vi "R5DOControl.vi"(8 "error constant":errorcluster, 11 "LabVIEW Web Service":refnum<class "Web Service.lvclass">) -> ()   [LabVIEW 2016]
uses:
  <vilib>/wsapi/Web Service.lvclass
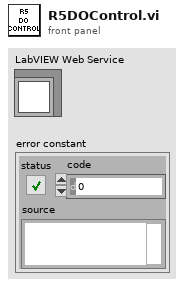
[diagram p1: front panel]
types:
  T1 = cluster{"DO Set Point":dbl, "Pump Time On, secs":dbl}
  T2 = cluster{"Signal, mA":dbl, "Value, UNITS HERE":dbl}
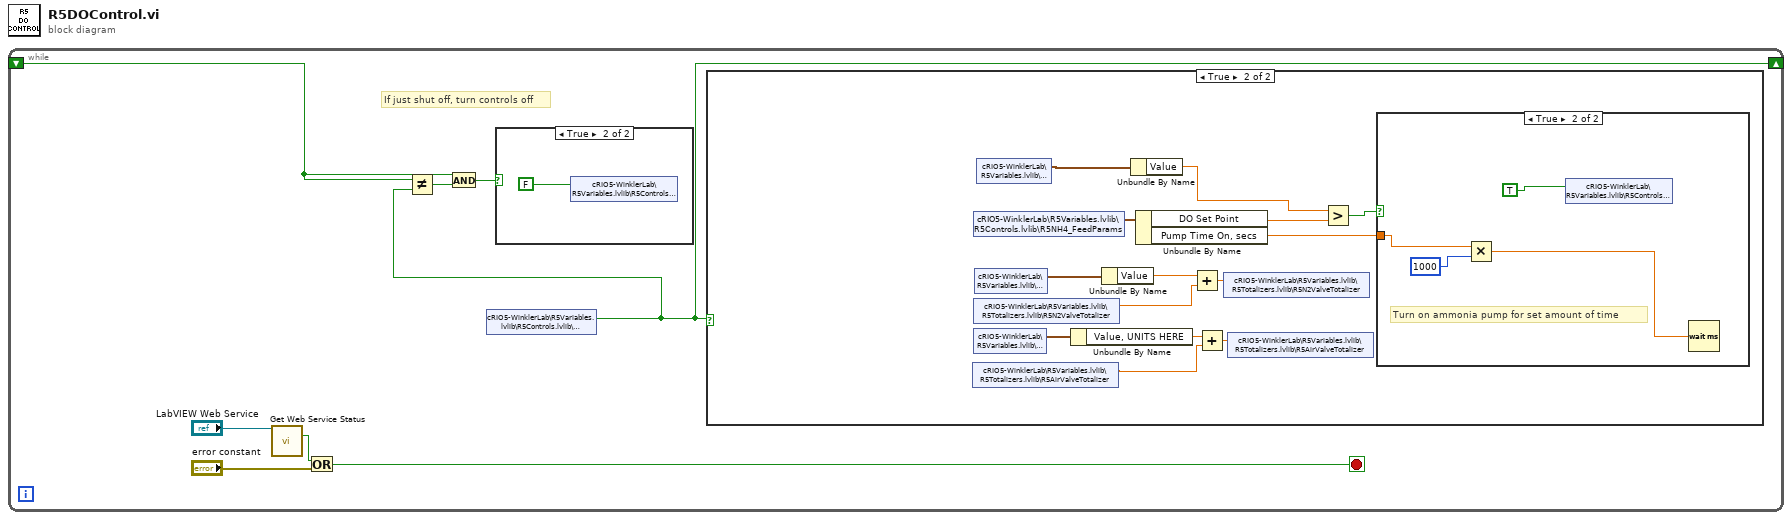
[diagram p0: block diagram]
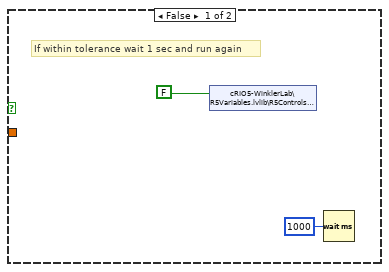
[diagram p4: hidden frame]
diagram:
  n1 = while {
    shift-right: [w1] -> _
    shift-left: _ -> [w2]
    stop <- w5 stop-if-true
    # "If just shut off, turn controls off"
    n2 = call <vilib>:"Get Web Service Status.vi"("LabVIEW Web Service"="LabVIEW Web Service") -> ("service stopping?"=w8:bool)  [unwired: 12 in, 2 out]
    n3 = Or(x=w8, y="error constant") -> (x .or. y?=w5:bool)
    n4 = shared-variable "cRIO5-WinklerLab\\R5Variables.lvlib\\R5Controls.lvlib\\R5DOSwitch"() -> (w1:bool)  [unwired: 1 in, 1 out]
    n5 = Not Equal?(x=w2, y=w1) -> (x != y?=w3:bool)
    n6 = And(x=w2, y=w3) -> (x .and. y?=w4:bool)
    n7 = case shown="True" w4 {
      frame False {
      }
      frame True {
        n8 = shared-variable "cRIO5-WinklerLab\\R5Variables.lvlib\\R5Controls.lvlib\\R5NH4Feed"(FALSE) -> ()  [unwired: 1 in, 1 out]
      }
    }
    n9 = case shown="True" w1 {
      frame False {
        # "Don't do anything if control is off"
      }
      frame True {
        n10 = shared-variable "cRIO5-WinklerLab\\R5Variables.lvlib\\R5Totalizers.lvlib\\R5AirValveTotalizer"() -> (w17:dbl)  [unwired: 1 in, 1 out]
        n11 = shared-variable "cRIO5-WinklerLab\\R5Variables.lvlib\\R5Controls.lvlib\\R5NH4_FeedParams"() -> (w13:T1)  [unwired: 1 in, 1 out]
        n12 = shared-variable "cRIO5-WinklerLab\\R5Variables.lvlib\\R5Totalizers.lvlib\\R5N2ValveTotalizer"() -> (w16:dbl)  [unwired: 1 in, 1 out]
        n13 = shared-variable "cRIO5-WinklerLab\\R5Variables.lvlib\\R5Signals.lvlib\\R5Air"() -> (w18:T2)  [unwired: 1 in, 1 out]
        n14 = shared-variable "cRIO5-WinklerLab\\R5Variables.lvlib\\R5Signals.lvlib\\R5N2"() -> (w19:cluster{"Signal":dbl, "Value":dbl})  [unwired: 1 in, 1 out]
        n15 = shared-variable "cRIO5-WinklerLab\\R5Variables.lvlib\\R5Signals.lvlib\\R5DO"() -> (w20:cluster{"Signal":dbl, "Value":dbl})  [unwired: 1 in, 1 out]
        n16 = Unbundle By Name(w18) -> ("Value, UNITS HERE"=w22:dbl)
        n17 = Unbundle By Name(w19) -> ("Value"=w21:dbl)
        n18 = Unbundle By Name(w20) -> ("Value"=w11:dbl)
        n19 = Unbundle By Name(w13) -> ("DO Set Point"=w12:dbl, "Pump Time On, secs"=w10:dbl)
        n20 = Add(x=w21, y=w16) -> (x+y=w15:dbl)
        n21 = Add(x=w22, y=w17) -> (x+y=w14:dbl)
        n22 = shared-variable "cRIO5-WinklerLab\\R5Variables.lvlib\\R5Totalizers.lvlib\\R5N2ValveTotalizer"(w15) -> ()  [unwired: 1 in, 1 out]
        n23 = shared-variable "cRIO5-WinklerLab\\R5Variables.lvlib\\R5Totalizers.lvlib\\R5AirValveTotalizer"(w14) -> ()  [unwired: 1 in, 1 out]
        n24 = Greater?(x=w11, y=w12) -> (0:w23:bool)
        n25 = case shown="True" w23 {
          tunnel: w10 -> [_ w28]
          frame False {
            # "If within tolerance wait 1 sec and run again"
            n26 = shared-variable "cRIO5-WinklerLab\\R5Variables.lvlib\\R5Controls.lvlib\\R5NH4Feed"(FALSE) -> ()  [unwired: 1 in, 1 out]
            n27 = Wait (ms)(milliseconds to wait=u32 1000) -> ()  [unwired: 1 out]
          }
          frame True {
            # "Turn on ammonia pump for set amount of time"
            n28 = Multiply(x=w28, y=1000) -> (x*y=w27:dbl)
            n29 = shared-variable "cRIO5-WinklerLab\\R5Variables.lvlib\\R5Controls.lvlib\\R5NH4Feed"(TRUE) -> ()  [unwired: 1 in, 1 out]
            n30 = Wait (ms)(milliseconds to wait=w27) -> ()  [unwired: 1 out]
          }
        }
      }
    }
  }
